vi "Autonomous Independent.vi"   [LabVIEW 2012]
doc: "This VI is called when autonomous begins, and will automatically be terminated when autonomous ends. You can carry out timed or sensor driven robot movement independently without needing to return to the caller."
uses:
  <vilib>/Rock Robotics/WPI/Solenoid/WPI_SolenoidValue.ctl
  Robot Global Data.vi
  <vilib>/Rock Robotics/WPI/Solenoid/WPI_SolenoidSetEnum.vi
  <vilib>/Rock Robotics/WPI/Joystick/WPI_JoystickGetSetRefNum.vi
panel:
  # "Be sure to right-click and choose Data Operations>>Make Current Value default if you want to save the array values with the VI"
types:
  T1 = typedef "WPI_JoystickDevRef.ctl" = cluster{"Device":T2}
  T2 = typedef "WPI_JoystickDeviceEnum.ctl" = enum16{"USB 1", "USB 2", "USB 3", "USB 4", "Kinect 1", "Kinect 2"}
  T3 = cluster{"axis 1 (x)":dbl, "axis 2 (y)":dbl, "axis 3 (throttle)":dbl, "axis 4":dbl, "axis 5":dbl, "axis 6":dbl}
  T4 = typedef "WPI_SolenoidValue.ctl" = enum16{"Off", "On", "Forward", "Reverse"}
  T5 = typedef "WPI_MotorControlDeviceRef.ctl" = cluster{"DeviceStatus":errorcluster, "Type":enum16{"PWM", "CAN"}, "PWM":cluster{"Digital Module":T6, "PWM Channel":T7, "DeadBand":T8}, "CAN":cluster{"Device Number":u8, "Control Mode":T9, "Semaphore":T10, "Max Vout":dbl}, "Invert":bool, "TransformRef":T11, "InvTransformRef":T11}
  T6 = typedef "FPGA_TypedefDigitalModule.ctl" = enum16{"Digital Module 1", "Digital Module 2"}
  T7 = typedef "FPGA_DIOPWMChannel.ctl" = enum8{"PWM 1", "PWM 2", "PWM 3", "PWM 4", "PWM 5", "PWM 6", "PWM 7", "PWM 8", "PWM 9", "PWM 10", "Invalid"}
  T8 = typedef "WPI_PWMDeadband.ctl" = cluster{"Name":string, "maxPositivePwm":i32, "minPositivePwm":i32, "centerPwm":i32, "maxNegativePwm":i32, "minNegativePwm":i32, "angularRange":u16}
  T9 = typedef "WPI_CANJaguar_ControlMode.ctl" = enum8{"Percent VBus", "Current", "Speed", "Position", "Voltage"}
  T10 = typedef "Semaphore RefNum" = refnum<k1>
  T11 = typedef "WPI_PWMTransform_ConPane.ctl" = refnum<vi>
  T12 = typedef "WPI_SolenoidDevRef.ctl" = cluster{"DevStatus":errorcluster, "Solenoid Module":T13, "Forward Solenoid Channel":T14, "Reverse Solenoid Channel":T14}
  T13 = typedef "FPGA_TypedefSolenoidModule.ctl" = enum16{"Solenoid Module 1", "Solenoid Module 2"}
  T14 = typedef "WPI_SolenoidChannel.ctl" = enum8{"Solenoid 1", "Solenoid 2", "Solenoid 3", "Solenoid 4", "Solenoid 5", "Solenoid 6", "Solenoid 7", "Solenoid 8", "Invalid"}
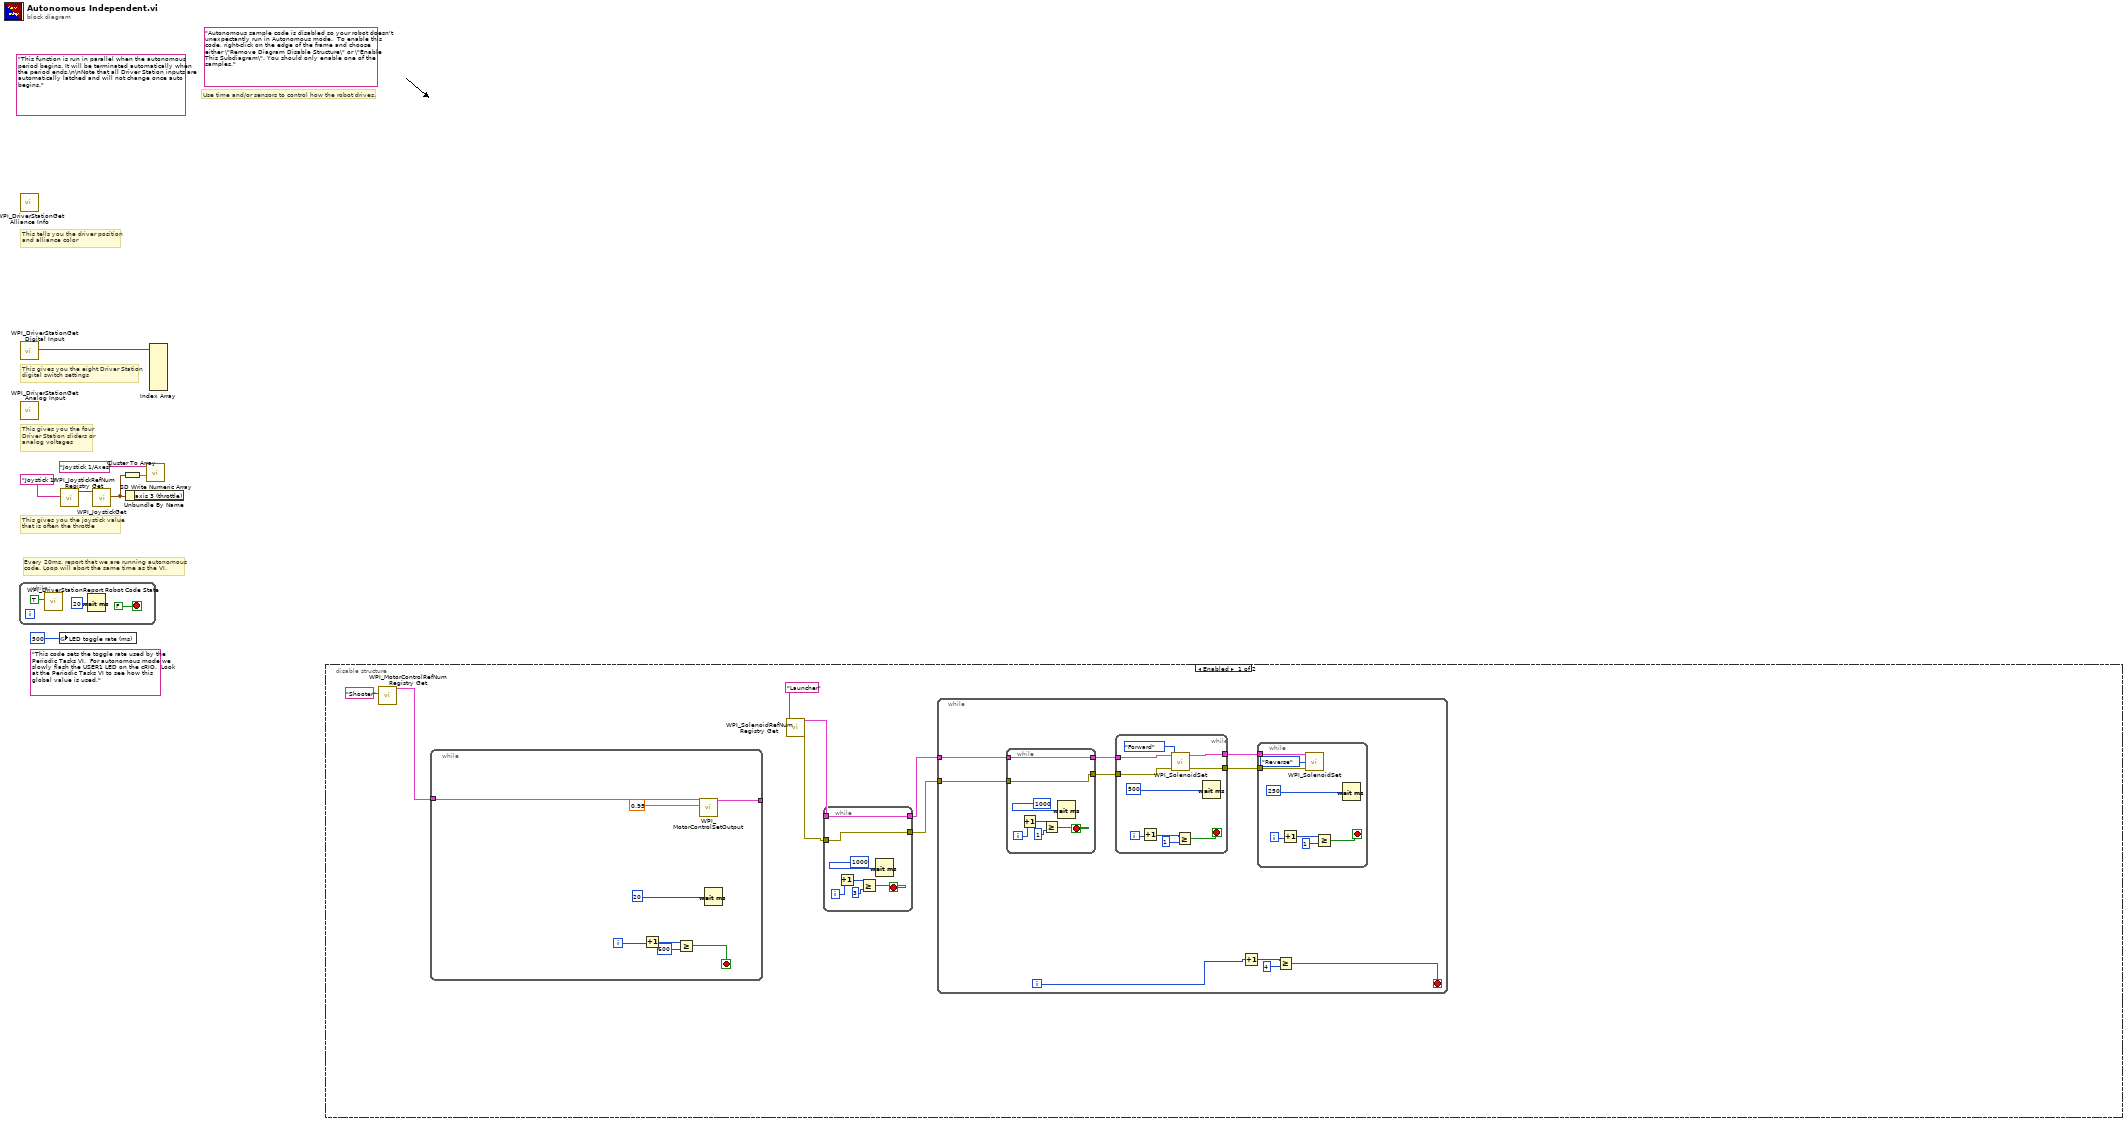
[diagram p0: block diagram]
diagram:
  (unwired) "This code sets the toggle rate used by the Periodic Tasks VI.  For autonomous mode we slowly flash the USER1 LED on the cRIO.  Look at the Periodic Tasks VI to see how this global value is used."
  (unwired) "Autonomous sample code is disabled so your robot doesn't unexpectantly run in Autonomous mode.  To enable this code, right-click on the edge of the frame and choose either \"Remove Diagram Disable Structure\" or \"Enable This Subdiagram\". You should only enable one of the samples."
  (unwired) "This function is run in parallel when the autonomous period begins. It will be terminated automatically when the period ends.\n\nNote that all Driver Station inputs are automatically latched and will not change once auto begins."
  # "Every 20ms, report that we are running autonomous\ncode. Loop will abort the same time as the VI."
  # "This gives you the joystick value\nthat is often the throttle"
  # "Use time and/or sensors to control how the robot drives."
  # "This tells you the driver position\nand alliance color"
  # "This gives you the eight Driver Station\ndigital switch settings"
  # "This gives you the four\nDriver Station sliders or\nanalog voltages"
  n1 = while {
    stop <- FALSE stop-if-true
    n2 = call <vilib>:"WPI_DriverStationReport Robot Code State.vi"("Autonomous"=TRUE) -> ()  [unwired: 10 in, 1 out]
    n3 = Wait (ms)(milliseconds to wait=u32 20) -> ()  [unwired: 1 out]
  }
  n4 = call <vilib>:"WPI_DriverStationGet Alliance Info.vi"() -> ()  [unwired: 12 out]
  n5 = call <vilib>:"WPI_DriverStationGet Digital Input.vi"() -> ("Driver Station Digital Input (1-8)"=w7:bool[])  [unwired: 11 out]
  n6 = call <vilib>:"WPI_DriverStationGet Analog Input.vi"() -> ()  [unwired: 12 out]
  n7 = global write "Robot Global Data.vi" "LED toggle rate (ms)"(u32 500 ("LED ms toggle rate")) -> ()
  n8 = call <vilib>:"WPI_JoystickRefNum Registry Get.vi"("refnum name"="Joystick 1") -> ("JoystickDevRef"=w5:T1)  [unwired: 1 in, 9 out]
  n9 = call <vilib>:"WPI_JoystickGet.vi"("JoystickDevRef"=w5) -> ("Axes"=w2:T3)  [unwired: 1 in, 5 out]
  n10 = Cluster To Array(cluster=w2) -> (array=w3:dbl[])
  n11 = Unbundle By Name(w2) -> ()  [unwired: 1 out]
  n12 = call <vilib>:"SD Write Numeric Array.vi"("Numeric Array"=w3, "Name"="Joystick 1/Axes") -> ()  [unwired: 8 in, 2 out]
  n13 = Index Array(array=w7) -> ()  [unwired: 8 in, 8 out]
  n14 = disable-structure shown="Enabled" {
    frame Enabled {
      n15 = call <vilib>:"WPI_MotorControlRefNum Registry Get.vi"("refnum name"="Shooter") -> ("MotorControlDevRef"=w17:T5)  [unwired: 9 in, 1 out]
      n16 = while {
        tunnel: w17 -> [w67]
        tunnel: [w60] -> _
        i -> [w64]
        stop <- w61 stop-if-true
        n17 = Increment(x=w64) -> (x+1=w63:i32)
        n18 = Greater Or Equal?(x=w63, y=600) -> (x >= y?=w61:bool)
        n19 = call <vilib>:"WPI_MotorControlSetOutput.vi"("Output"=0.95, "MotorControlDevRef"=w67) -> ("MotorControlDevRef"=w60:T5)  [unwired: 7 in, 2 out]
        n20 = Wait (ms)(milliseconds to wait=u32 20) -> ()  [unwired: 1 out]
      }
      n21 = call <vilib>:"WPI_SolenoidRefNum Registry Get.vi"("refnum name"="Launcher") -> ("error out"=w14:errorcluster, "SolenoidDevRef"=w13:T12)  [unwired: 9 in]
      n22 = while {
        tunnel: [w19] -> w12
        tunnel: w13 -> [w19]
        tunnel: [w18] -> _
        tunnel: w14 -> [w18]
        tunnel: [w18] -> w11
        i -> [w20]
        stop <- w21 stop-if-true
        n23 = Increment(x=w20) -> (x+1=w23:i32)
        n24 = Greater Or Equal?(x=w23, y=3) -> (x >= y?=w21:bool)
        n25 = Wait (ms)(milliseconds to wait=u32 1000) -> ()  [unwired: 1 out]
      }
      n26 = while {
        tunnel: w12 -> [w28]
        tunnel: w11 -> [w26]
        i -> [w31]
        stop <- w32 stop-if-true
        n27 = while {
          tunnel: [w36] -> w29
          tunnel: w28 -> [w36]
          tunnel: [w35] -> w27
          tunnel: w26 -> [w35]
          i -> [w37]
          stop <- w38 stop-if-true
          n28 = Increment(x=w37) -> (x+1=w40:i32)
          n29 = Greater Or Equal?(x=w40, y=1) -> (x >= y?=w38:bool)
          n30 = Wait (ms)(milliseconds to wait=u32 1000) -> ()  [unwired: 1 out]
        }
        n31 = while {
          tunnel: [w54] -> w30
          tunnel: w29 -> [w53]
          tunnel: w27 -> [w52]
          tunnel: [w51] -> w25
          i -> [w55]
          stop <- w56 stop-if-true
          n32 = Increment(x=w55) -> (x+1=w58:i32)
          n33 = call-poly <vilib>:"WPI_SolenoidSet.vi"("error in (no error)"=w52, "Value"=WPI_SolenoidValue."Forward", "SolenoidDevRef"=w53) -> ("error out"=w51:errorcluster, "SolenoidDevRef"=w54:T12)  [unwired: 7 in]
          n34 = Greater Or Equal?(x=w58, y=1) -> (x >= y?=w56:bool)
          n35 = Wait (ms)(milliseconds to wait=u32 500) -> ()  [unwired: 1 out]
        }
        n36 = Increment(x=w31) -> (x+1=w34:i32)
        n37 = while {
          tunnel: w30 -> [w44]
          tunnel: w25 -> [w43]
          i -> [w45]
          stop <- w46 stop-if-true
          n38 = Increment(x=w45) -> (x+1=w48:i32)
          n39 = call-poly <vilib>:"WPI_SolenoidSet.vi"("error in (no error)"=w43, "Value"=WPI_SolenoidValue."Reverse", "SolenoidDevRef"=w44) -> ()  [unwired: 7 in, 2 out]
          n40 = Greater Or Equal?(x=w48, y=1) -> (x >= y?=w46:bool)
          n41 = Wait (ms)(milliseconds to wait=u32 250) -> ()  [unwired: 1 out]
        }
        n42 = Greater Or Equal?(x=w34, y=4) -> (x >= y?=w32:bool)
      }
    }
    frame Disabled {
    }
  }
